vi "alt change indicator.vi"(4 "Cluster":cluster{"x":i32, "y":i32}={"x"=25, "y"=32}, 6 "size":i16=29, 7 "change":dbl(slide) scale=-2.0..2.0, 10 "pict in":picture) -> (3 "pict out":picture)   [LabVIEW 2017]
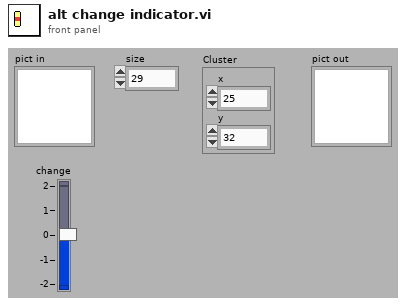
[diagram p1: front panel]
types:
  T1 = cluster{"left":i16, "top":i16, "right":i16, "bottom":i16}
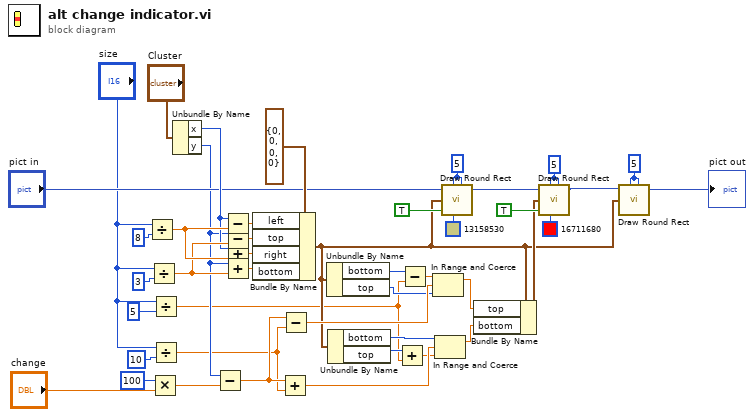
[diagram p0: block diagram]
diagram:
  w10 = i16 5 ("oval height")
  w23 = i16 5 ("oval height")
  w36 = i16 5 ("oval height")
  n1 = Divide(x="size", y=i16 8) -> (x/y=w33:dbl)
  n2 = Divide(x="size", y=i16 3) -> (x/y=w30:dbl)
  n3 = Multiply(x=100, y="change") -> (x*y=w42:dbl)
  n4 = Divide(x="size", y=i16 5) -> (x/y=w2:dbl)
  n5 = Divide(x="size", y=10) -> (x/y=w4:dbl)
  n6 = Unbundle By Name("Cluster") -> ("x"=w28:i32, "y"=w11:i32)
  n7 = Subtract(x=w11, y=w42) -> (x-y=w15:dbl)
  n8 = Subtract(x=w28, y=w33) -> (x-y=w27:dbl)
  n9 = Subtract(x=w11, y=w30) -> (x-y=w37:dbl)
  n10 = Add(x=w28, y=w33) -> (x+y=w35:dbl)
  n11 = Add(x=w11, y=w30) -> (x+y=w34:dbl)
  n12 = Bundle By Name(cluster=T1 {"left"=0, "top"=0, "right"=0, "bottom"=0} ("rect"), "left"=w27, "top"=w37, "right"=w35, "bottom"=w34) -> (w12:T1)
  n13 = Add(x=w15, y=w4) -> (x+y=w16:dbl)
  n14 = Subtract(x=w15, y=w4) -> (x-y=w17:dbl)
  n15 = Unbundle By Name(w12) -> ("bottom"=w7:i16, "top"=w9:i16)
  n16 = Unbundle By Name(w12) -> ("bottom"=w13:i16, "top"=w14:i16)
  n17 = Add(x=w14, y=w2) -> (x+y=w3:dbl)
  n18 = Subtract(x=w7, y=w2) -> (x-y=w8:dbl)
  n19 = In Range and Coerce(upper limit=w8, x=w17, lower limit=w9) -> (coerced(x)=w1:dbl)  [unwired: 1 out]
  n20 = In Range and Coerce(upper limit=w13, x=w16, lower limit=w3) -> (coerced(x)=w18:dbl)  [unwired: 1 out]
  n21 = call <vilib>:"Draw Round Rect.vi"("picture"="pict in", "oval width"=w36, "rect"=w12, "fill?(F)"=TRUE, "color(black)"=u32 13158530 ("color sky"), "oval height"=w36) -> ("new picture"=w25:picture)  [unwired: 3 in]
  n22 = Bundle By Name(cluster=w12, "top"=w1, "bottom"=w18) -> (w20:T1)
  n23 = call <vilib>:"Draw Round Rect.vi"("picture"=w25, "oval width"=w10, "rect"=w20, "fill?(F)"=TRUE, "color(black)"=u32 16711680 ("color gound"), "oval height"=w10) -> ("new picture"=w19:picture)  [unwired: 3 in]
  n24 = call <vilib>:"Draw Round Rect.vi"("picture"=w19, "oval width"=w23, "rect"=w12, "oval height"=w23) -> ("new picture"=→"pict out":picture)  [unwired: 5 in]
